vi "startSALMonitor.vi"(8 "error in (no error)":errorcluster, 10 "Component":string, 11 "SystemSettings in":refnum<class "SystemSettings.lvclass">) -> (0 "error out":errorcluster, 3 "SystemSettings out":refnum<class "SystemSettings.lvclass">)   [LabVIEW 2016, in "SystemSettings.lvclass"]
uses:
  SystemSettings.lvclass
panel:
  out "return code":i32
  out "standard error":string
  out "standard output":string
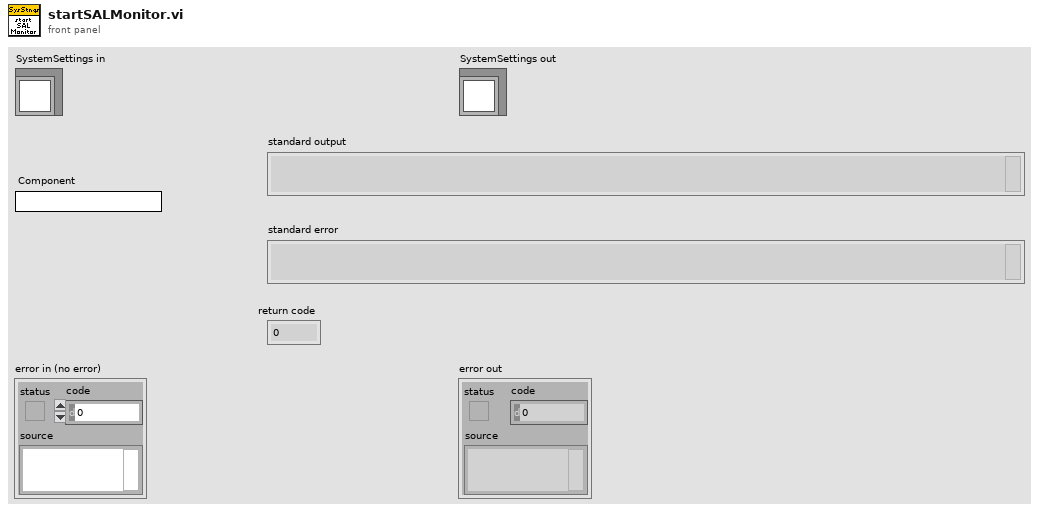
[diagram p1: front panel]
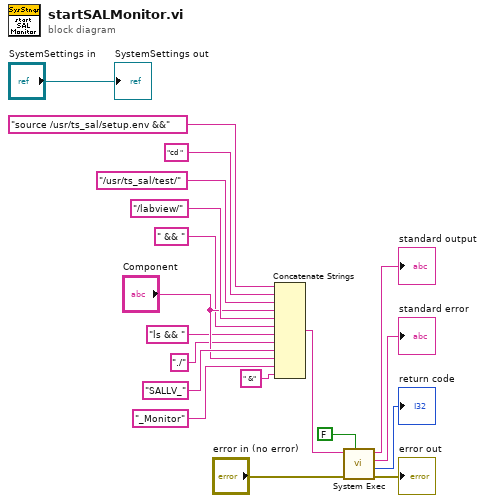
[diagram p0: block diagram]
diagram:
  n1 = Concatenate Strings("source /usr/ts_sal/setup.env &&" ("command line"), "cd " ("string"), "/usr/ts_sal/test/" ("string"), "Component", "/labview/" ("string"), " && " ("string"), "ls && " ("string"), "./" ("string"), "SALLV_" ("string"), "Component", "_Monitor" ("string"), " &" ("string")) -> (w12:string)
  n2 = call <vilib>:"System Exec.vi"("wait until completion? (T)"=FALSE, "error in (no error)"="error in (no error)", "command line"=w12) -> ("error out"=→"error out":errorcluster, "return code"=→"return code":i32, "standard error"=→"standard error":string, "standard output"=→"standard output":string)  [unwired: 5 in]
  "SystemSettings out" <- "SystemSettings in"
